vi "Sweep_Ctrl.vi"(8 "error in (no error)":errorcluster, 9 "Stop_freq [Hz]":ext=40.0, 10 "Step_freq [Hz]":ext=5.0, 11 "Start_freq [Hz]":ext=40.0) -> (0 "error out":errorcluster, 2 "Inv_Freq_Array":ext[](array[numeric]), 3 "Freq_Array":ext[](array[numeric]))   [LabVIEW 2017]
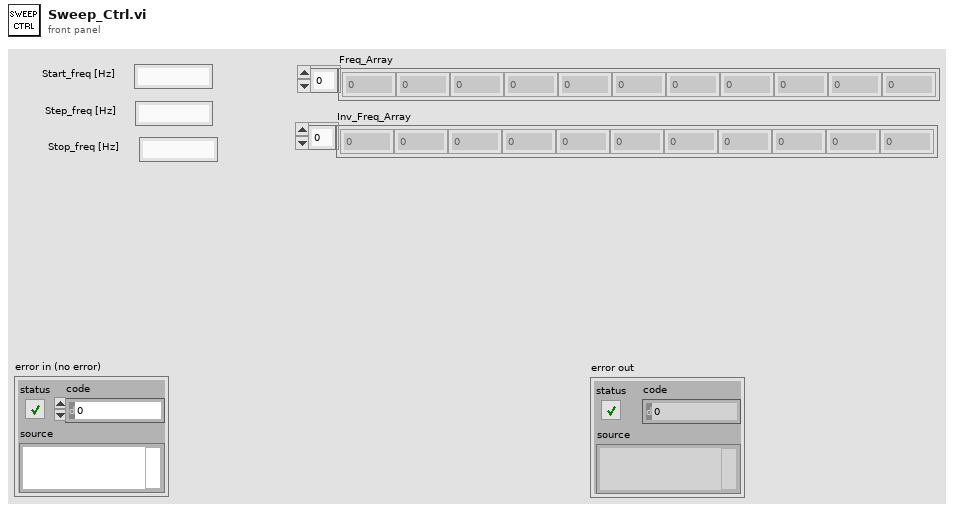
[diagram p1: front panel]
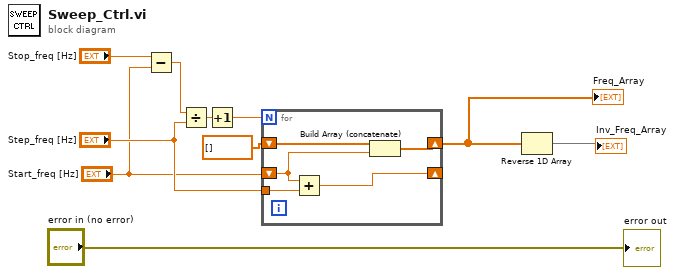
[diagram p0: block diagram]
diagram:
  n1 = Subtract(x="Stop_freq [Hz]", y="Start_freq [Hz]") -> (x-y=w4:ext)
  n2 = Divide(x=w4, y="Step_freq [Hz]") -> (x/y=w7:ext)
  n3 = Increment(x=w7) -> (x+1=w8:ext)
  n4 = for {
    N: w8 -> [_]
    tunnel: "Step_freq [Hz]" -> [w15]
    shift-right: [w13] -> w2
    shift-left: ext[] [] -> [w12]
    shift-right: [w14] -> _
    shift-left: "Start_freq [Hz]" -> [w11]
    n5 = Add(x=w11, y=w15) -> (x+y=w14:ext)
    n6 = Build Array (concatenate)(w12, w11) -> (w13:ext[])
  }
  "Freq_Array" <- w2
  n7 = Reverse 1D Array(array=w2) -> (reversed array=→"Inv_Freq_Array":ext[])
  "error out" <- "error in (no error)"
